vi "purge_nozzle.vi"(4 "purge frequency":dbl, 5 "Purge":bool) -> ()   [LabVIEW 2011]
doc: "enables or disables the nozzle purge mode for the Trigger"
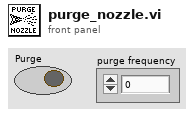
[diagram p1: front panel]
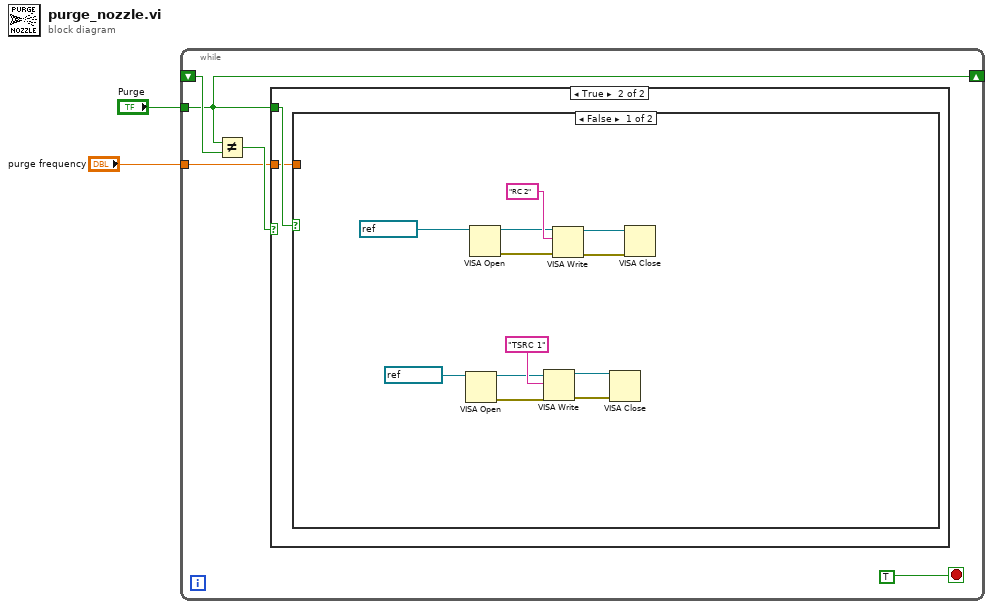
[diagram p0: block diagram]
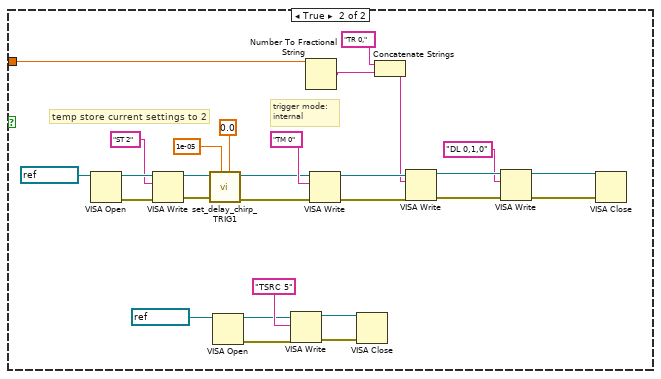
[diagram p3: hidden frame]
diagram:
  n1 = while {
    shift-right: [w4] -> _
    shift-left: _ -> [w7]
    tunnel: "Purge" -> [w4]
    tunnel: "purge frequency" -> [w3]
    stop <- TRUE stop-if-true
    n2 = Not Equal?(x=w4, y=w7) -> (x != y?=w6:bool)
    n3 = case shown="True" w6 {
      tunnel: w4 -> [_ w9]
      tunnel: w3 -> [_ w8]
      frame False {
      }
      frame True {
        n4 = case shown="False" w9 {
          tunnel: w8 -> [_ w28]
          frame False {
            n5 = VISA Open(VISA resource name=refnum<visa-resource-name> "TRIG2") -> (VISA resource name=w14:refnum<visa-resource-name>, error out=w13:errorcluster)  [unwired: 4 in]
            n6 = VISA Open(VISA resource name=refnum<visa-resource-name> "TRIG1") -> (VISA resource name=w19:refnum<visa-resource-name>, error out=w18:errorcluster)  [unwired: 4 in]
            n7 = VISA Write(VISA resource name=w14, write buffer="TSRC 1" ("Query 2"), error in (no error)=w13) -> (VISA resource name out=w11:refnum<visa-resource-name>, error out=w10:errorcluster)  [unwired: 1 out]
            n8 = VISA Write(VISA resource name=w19, write buffer="RC 2", error in (no error)=w18) -> (VISA resource name out=w17:refnum<visa-resource-name>, error out=w16:errorcluster)  [unwired: 1 out]
            n9 = VISA Close(VISA resource name=w11, error in (no error)=w10) -> ()  [unwired: 1 out]
            n10 = VISA Close(VISA resource name=w17, error in (no error)=w16) -> ()  [unwired: 1 out]
          }
          frame True {
            # "trigger mode:\ninternal"
            # "temp store current settings to 2"
            n11 = VISA Open(VISA resource name=refnum<visa-resource-name> "TRIG1") -> (VISA resource name=w37:refnum<visa-resource-name>, error out=w48:errorcluster)  [unwired: 4 in]
            n12 = VISA Write(VISA resource name=w37, write buffer="ST 2", error in (no error)=w48) -> (VISA resource name out=w35:refnum<visa-resource-name>, error out=w34:errorcluster)  [unwired: 1 out]
            n13 = call "set_delay_chirp_TRIG1.vi"("background period"=0.0, "inhibit off"=1e-05 ("molecular delay"), "error in"=w34, "VISA resource name"=w35) -> ("error out"=w43:errorcluster, "VISA resource name out"=w44:refnum<visa-resource-name>)  [unwired: 6 in]
            n14 = VISA Open(VISA resource name=refnum<visa-resource-name> "TRIG2") -> (VISA resource name=w26:refnum<visa-resource-name>, error out=w25:errorcluster)  [unwired: 4 in]
            n15 = VISA Write(VISA resource name=w26, write buffer="TSRC 5" ("Query 2"), error in (no error)=w25) -> (VISA resource name out=w23:refnum<visa-resource-name>, error out=w22:errorcluster)  [unwired: 1 out]
            n16 = Number To Fractional String(number=w28) -> (F-format string=w29:string)  [unwired: 3 in]
            n17 = VISA Write(VISA resource name=w44, write buffer="TM 0", error in (no error)=w43) -> (VISA resource name out=w42:refnum<visa-resource-name>, error out=w41:errorcluster)  [unwired: 1 out]
            n18 = VISA Close(VISA resource name=w23, error in (no error)=w22) -> ()  [unwired: 1 out]
            n19 = Concatenate Strings("TR 0," ("string"), w29) -> (w38:string)
            n20 = VISA Write(VISA resource name=w42, write buffer=w38, error in (no error)=w41) -> (VISA resource name out=w32:refnum<visa-resource-name>, error out=w40:errorcluster)  [unwired: 1 out]
            n21 = VISA Write(VISA resource name=w32, write buffer="DL 0,1,0", error in (no error)=w40) -> (VISA resource name out=w31:refnum<visa-resource-name>, error out=w33:errorcluster)  [unwired: 1 out]
            n22 = VISA Close(VISA resource name=w31, error in (no error)=w33) -> ()  [unwired: 1 out]
          }
        }
      }
    }
  }
